vi "UI.Stream.Disable.vi"(8 "error in (no error)":errorcluster, 11 "State Variables in":T1) -> (0 "error out":errorcluster)   [LabVIEW 2019, in "J1939 Workspace Shared.lvlib"]
uses:
  J1939 Workspace Shared.lvlib
  Types/UI.StateVariables.ctl
  <vilib>/NI VeriStand/Display Template Support/DisplayTemplateSupport.llb/enum_Display Template Handler Minimal To Widget Msg.ctl
  <vilib>/NI VeriStand/Execution/Workspace/SystemStateRegEventRef.ctl
  <vilib>/NI VeriStand/Execution/Workspace/Target State Info.ctl
  <vilib>/NI VeriStand/Execution/Workspace/Target State.ctl
  Types/Private Data.ctl
  <vilib>/NI/STM/TCP/TCP Connection Info.ctl
  <vilib>/NI/STM/SubVIs/MetaDataElement.ctl
  Addon/Addon Shared/Types/Error Cluster.ctl
  Addon/Addon Shared/Types/Error Types.ctl
  NationalInstruments.VeriStand.SystemStorage
  <vilib>/NI VeriStand/Display Template Support/DisplayTemplateSupport.llb/enum_Display Template Handler Minimal To Workspace.ctl
  <vilib>/NI VeriStand/Execution/Workspace/WorkspaceAPI.ctl
  NationalInstruments.VeriStand.ClientAPI
  <vilib>/NI VeriStand/Execution/Workspace/SystemStateEventRef.ctl
  Types/UI.Refs.ctl
  SubModules/CAN-Streaming-Support/Addon/Addon Shared/Types/Type Filter.ctl
  SubModules/CAN-Streaming-Support/Addon/Addon Shared/Types/Direction Filter.ctl
  SubModules/CAN-Streaming-Support/UIs/Workspace Shared/Types/Host Stream Queue Refs.ctl
  SubModules/CAN-Streaming-Support/UIs/Workspace Shared/Types/Host Stream Queue Type.ctl
  SubModules/CAN-Streaming-Support/UIs/Workspace Shared/Types/Host Stream Queue Command.ctl
  <vilib>/xnet/xnet.llb/XNET Frame CAN.ctl
  <vilib>/xnet/xnet.llb/XNET Frame Type CAN.ctl
  <vilib>/Utility/miscctls.llb/LVRowAndColumnUnsignedTypeDef.ctl
  <vilib>/NI VeriStand/Execution/Workspace/NI_VS Workspace ExecutionAPI.lvlib
  SubModules/CAN-Streaming-Support/UIs/Workspace Shared/CAN Stream Support Workspace Shared.lvlib
  SubModules/CAN-Streaming-Support/Addon/Addon Shared/CAN Stream Support Shared.lvlib
  Addon/Addon Shared/J1939 Addon Shared.lvlib
  <vilib>/NI/STM/NI STM.lvlib
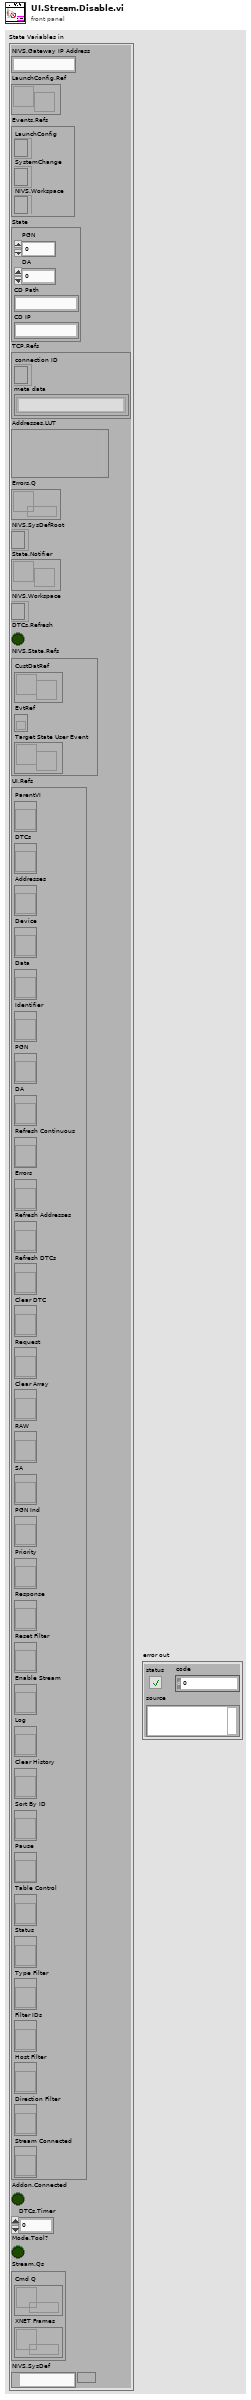
[diagram p1: front panel]
types:
  T1 = typedef "J1939 Workspace Shared.lvlib/UI.StateVariables.ctl" = cluster{"NIVS.Gateway IP Address":string, "LaunchConfig.Ref":refnum<user-event>, "Events.Refs":cluster{"LaunchConfig":refnum<event-registration>, "SystemChange":T2, "NIVS.Workspace":refnum<event-registration>}, "State":T3, "TCP.Refs":T4, "Addresses.LUT":variant, "Errors.Q":refnum<queue>, "NIVS.SysDefRoot":refnum<k24>, "State.Notifier":refnum<user-event>, "NIVS.Workspace":T6, "DTCs.Refresh":bool, "NIVS.State.Refs":T7, "UI.Refs":T8, "Addon.Connected":bool, "DTCs.Timer":u32, "Mode.Tool?":bool, "Stream.Qs":T9, "NIVS.SysDef":path}
  T2 = typedef "NI_VS Workspace ExecutionAPI.lvlib/SystemStateRegEventRef.ctl" = refnum<event-registration>
  T3 = typedef "J1939 Workspace Shared.lvlib/Private Data.ctl" = cluster{"PGN":u32, "DA":u8, "CD Path":string, "CD IP":string}
  T4 = typedef "NI STM.lvlib/TCP Connection Info.ctl" = cluster{"connection ID":refnum<k5>, "meta data":T5[]}
  T5 = typedef "NI STM.lvlib/MetaDataElement.ctl" = string
  T6 = typedef "NI_VS Workspace ExecutionAPI.lvlib/WorkspaceAPI.ctl" = refnum<k24>
  T7 = typedef "NI_VS Workspace ExecutionAPI.lvlib/SystemStateEventRef.ctl" = cluster{"CustDatRef":refnum<user-event>, "EvtRef":refnum<k27>, "Target State User Event":refnum<user-event>}
  T8 = typedef "J1939 Workspace Shared.lvlib/UI.Refs.ctl" = cluster{"ParentVI":refnum<vi>, "DTCs":refnum<vi>, "Addresses":refnum<vi>, "Device":refnum<vi>, "Data":refnum<vi>, "Identifier":refnum<vi>, "PGN":refnum<vi>, "DA":refnum<vi>, "Refresh Continuous":refnum<vi>, "Errors":refnum<vi>, "Refresh Addresses":refnum<vi>, "Refresh DTCs":refnum<vi>, "Clear DTC":refnum<vi>, "Request":refnum<vi>, "Clear Array":refnum<vi>, "RAW":refnum<vi>, "SA":refnum<vi>, "PGN Ind":refnum<vi>, "Priority":refnum<vi>, "Response":refnum<vi>, "Reset Filter":refnum<vi>, "Enable Stream":refnum<vi>, "Log":refnum<vi>, "Clear History":refnum<vi>, "Sort By ID":refnum<vi>, "Pause":refnum<vi>, "Table Control":refnum<vi>, "Status":refnum<vi>, "Type Filter":refnum<vi>, "Filter IDs":refnum<vi>, "Host Filter":refnum<vi>, "Direction Filter":refnum<vi>, "Stream Connected":refnum<vi>}
  T9 = typedef "CAN Stream Support Workspace Shared.lvlib/Host Stream Queue Refs.ctl" = cluster{"Cmd Q":refnum<queue>, "XNET Frames":refnum<queue>}
  T10 = typedef "LVRowAndColumnUnsignedTypeDef.ctl" = cluster{"Row":u32, "Column":u32}
  T11 = enum8{"Enabled", "Disabled", "Disabled and Grayed Out"}
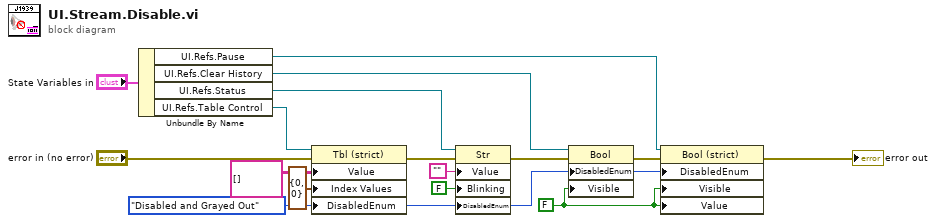
[diagram p0: block diagram]
diagram:
  w2 = FALSE ("Value")
  w3 = T11."Disabled and Grayed Out" ("Disabled")
  n1 = Unbundle By Name("State Variables in") -> ("UI.Refs.Pause"=w4:refnum<vi>, "UI.Refs.Clear History"=w8:refnum<vi>, "UI.Refs.Status"=w13:refnum<vi>, "UI.Refs.Table Control"=w15:refnum<vi>)
  n2 = property class="Tbl (strict)"(reference=w15, error in="error in (no error)", "Value"=string[][] [], "Index Values"=T10 {"Row"=0, "Column"=0}, "DisabledEnum"=w3) -> (error out=w9:errorcluster)  [unwired: 1 out]
  n3 = property class="Str"(reference=w13, error in=w9, "Value"="", "Blinking"=FALSE, "DisabledEnum"=w3) -> (error out=w7:errorcluster)  [unwired: 1 out]
  n4 = property class="Bool"(reference=w8, error in=w7, "DisabledEnum"=w3, "Visible"=w2) -> (error out=w5:errorcluster)  [unwired: 1 out]
  n5 = property class="Bool (strict)"(reference=w4, error in=w5, "DisabledEnum"=w3, "Visible"=w2, "Value"=w2) -> (error out=→"error out":errorcluster)  [unwired: 1 out]
